vi "Configure Step.vi"(0 "VISA resource name":refnum<visa-resource-name>, 1 "Output AC Voltage Frequency (60  Hz)":dbl=60.0 min=45.0 max=500.0 format="%.1p", 2 "Output AC Voltage (115 V)":dbl=115.0 min=0.0 max=300.0 format="%.1f", 3 "Step Prompt":T1={"Enable Prompt"=FALSE, "Prompt ( )"=" "}, 5 "Step (1)":i32=1 min=1 max=9 step=1, 7 "Step Cycle (1)":i32=1 min=0 max=9999 step=1, 9 "Enable Step Connection (F:Disable)":bool, 11 "error in (no error)":errorcluster, 12 "Voltage Range Mode (1:Auto)":u16(ring)=1 items=["High", "Auto"], 13 "Start Angle (0)":i32 min=0 max=359, 14 "End Angle: (0)":i32 min=0 max=359) -> (4 "VISA resource name out":refnum<visa-resource-name>, 15 "error out":errorcluster)   [LabVIEW 2020, in "eec 6700.lvlib"]
doc: "Configures the user specified step and its parameters in the current Memory location (Use \"Configure Memory.vi\" to select the desired memory)\n\nNote : Run \"Configure Program Mode.vi\" to make sure the instrument is in <B>Program Mode</B> before using this VI"
uses:
  <instrlib>/eec 6700/eec 6700.lvlib
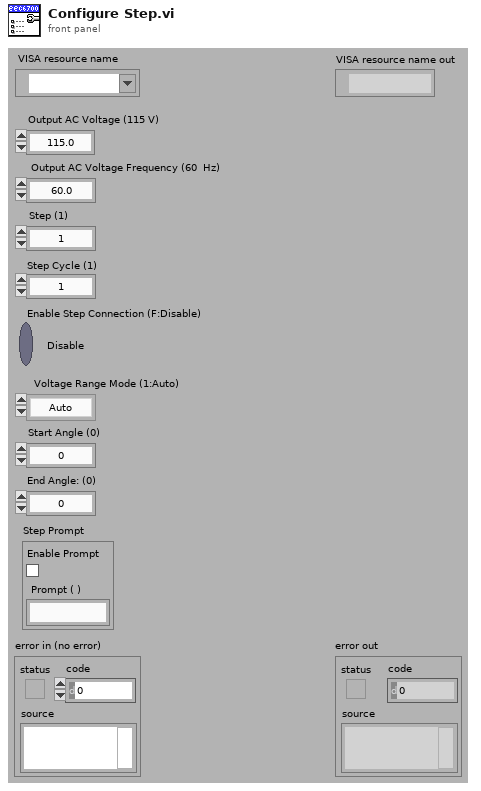
[diagram p1: front panel]
types:
  T1 = cluster{"Enable Prompt":bool, "Prompt ( )":string}
  T2 = typedef "eec 6700.lvlib/Extended User Data.ctl" = cluster{"Firmware Version":string, "eec Models":enum16{"6605", "6610", "6620", "6630", "6650"}}
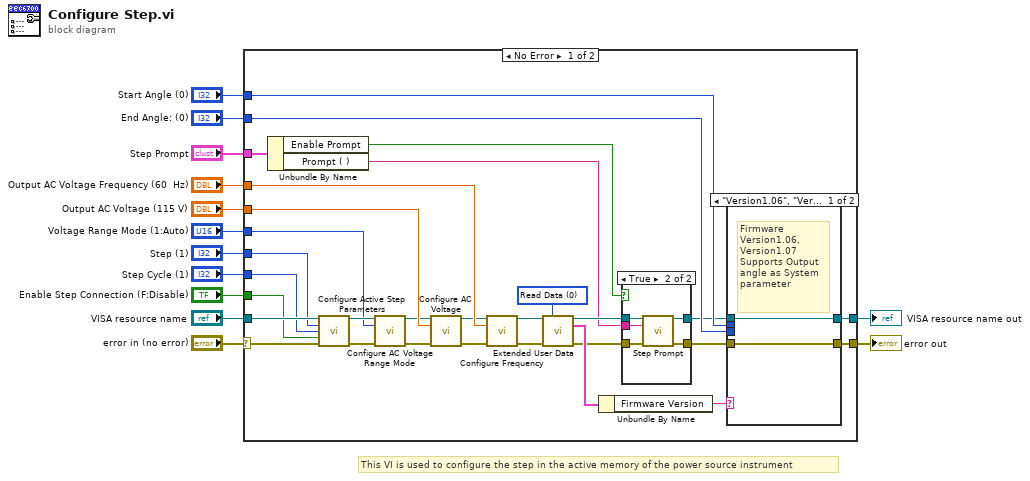
[diagram p0: block diagram]
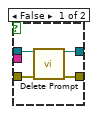
[diagram p2: hidden frame]
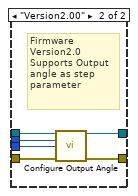
[diagram p3: hidden frame]
diagram:
  # "This VI is used to configure the step in the active memory of the power source instrument"
  n1 = case shown="No Error" "error in (no error)" {
    selector: "error in (no error)" -> [w42 w62]
    tunnel: [w29 w62] -> w13
    tunnel: [w30 w61] -> w12
    tunnel: "VISA resource name" -> [w43 w61]
    tunnel: "Output AC Voltage Frequency (60  Hz)" -> [w41 _]
    tunnel: "Step Cycle (1)" -> [w40 _]
    tunnel: "Enable Step Connection (F:Disable)" -> [w39 _]
    tunnel: "Step (1)" -> [w38 _]
    tunnel: "Output AC Voltage (115 V)" -> [w32 _]
    tunnel: "Voltage Range Mode (1:Auto)" -> [w31 _]
    tunnel: "Start Angle (0)" -> [w23 _]
    tunnel: "End Angle: (0)" -> [w22 _]
    tunnel: "Step Prompt" -> [w17 _]
    frame No Error {
      w26 = u16 0 items=["Read Data", "Write Data", "Clear Data", "Clear ALL Data"] ("Action")
      n2 = Unbundle By Name(w17) -> ("Enable Prompt"=w15:bool, "Prompt ( )"=w16:string)
      n3 = call <instrlib>:"Configure Active Step Parameters.vi"("VISA resource name"=w43, "Step (1)"=w38, "Step Cycle (1)"=w40, "Enable Step Connection (F:Disable)"=w39, "error in (no error)"=w42) -> ("VISA resource name out"=w37:refnum<visa-resource-name>, "error out"=w36:errorcluster)  [unwired: 9 in]
      n4 = call <instrlib>:"Configure AC Voltage Range Mode.vi"("VISA resource name"=w37, "Voltage Range Mode (1:Auto)"=w31, "error in (no error)"=w36) -> ("VISA resource name out"=w14:refnum<visa-resource-name>, "error out"=w35:errorcluster)  [unwired: 11 in]
      n5 = call <instrlib>:"Configure AC Voltage.vi"("VISA resource name"=w14, "Output AC Voltage (115 V)"=w32, "error in (no error)"=w35) -> ("VISA resource name out"=w33:refnum<visa-resource-name>, "error out"=w34:errorcluster)  [unwired: 11 in]
      n6 = call <instrlib>:"Configure Frequency.vi"("VISA resource name"=w33, "Output AC Voltage Frequency (60  Hz)"=w41, "error in (no error)"=w34) -> ("VISA resource name out"=w27:refnum<visa-resource-name>, "error out"=w28:errorcluster)  [unwired: 11 in]
      n7 = call <instrlib>:"Extended User Data.vi"("VISA resource name"=w27, "Action"=w26, "Error In (no error)"=w28) -> ("VISA resource name out"=w21:refnum<visa-resource-name>, "User Data Out"=w25:T2, "Error Out"=w19:errorcluster)  [unwired: 10 in]
      n8 = Unbundle By Name(w25) -> ("Firmware Version"=w24:string)
      n9 = case shown="True" w15 {
        tunnel: w21 -> [w47 w52]
        tunnel: [w45 w51] -> w20
        tunnel: w19 -> [w44 w50]
        tunnel: [w46 w49] -> w18
        tunnel: w16 -> [_ w48]
        frame False {
          n10 = call <instrlib>:"Delete Prompt.vi"("VISA resource name"=w47, "error in (no error)"=w44) -> ("VISA resource name out"=w45:refnum<visa-resource-name>, "error out"=w46:errorcluster)  [unwired: 12 in]
        }
        frame True {
          n11 = call <instrlib>:"Step Prompt.vi"("VISA resource name"=w52, "Prompt ( )"=w48, "error in (no error)"=w50) -> ("VISA resource name out"=w51:refnum<visa-resource-name>, "error out"=w49:errorcluster)  [unwired: 11 in]
        }
      }
      n12 = case shown="\"Version1.06\", \"Version1.07\", Default" w24 {
        tunnel: [w54 w60] -> w30
        tunnel: [w53 w59] -> w29
        tunnel: w18 -> [w53 w58]
        tunnel: w20 -> [w54 w57]
        tunnel: w23 -> [_ w56]
        tunnel: w22 -> [_ w55]
        frame "Version1.06", "Version1.07", Default {
          # "Firmware \nVersion1.06,\nVersion1.07\nSupports Output\nangle as System\nparameter"
        }
        frame "Version2.00" {
          # "Firmware \nVersion2.0\nSupports Output\nangle as step\nparameter"
          n13 = call <instrlib>:"Configure Output Angle.vi"("VISA resource name"=w57, "Start Angle (0)"=w56, "End Angle: (0)"=w55, "error in (no error)"=w58) -> ("VISA resource name out"=w60:refnum<visa-resource-name>, "error out"=w59:errorcluster)  [unwired: 10 in]
        }
      }
    }
    frame Error {
    }
  }
  "error out" <- w13
  "VISA resource name out" <- w12
